vi "FdxCmdRxUDPControlCvi.vi"(8 "error in":errorcluster, 9 "UdpControl":T1={"UdpHandle"=0, "NetSelect"=3, "InterruptControl"=0} {"NetSelect" items=["FDX_RX_UDP_ONLY_A"=1, "FDX_RX_UDP_ONLY_B"=2, "FDX_RX_UDP_BOTH"=3]}, 11 "InstrumentHandle_port":u32) -> (0 "error out":errorcluster, 3 "InstrumentHandle_port":u32)   [LabVIEW 2020, in "AIM664LV.lvlib"]
doc: "This function allows to configure several settings of a UDP Receive Port"
uses:
  AIM664LV.lvlib
  AFDX_LibraryAdmin/FdxGlobalDllPath.vi
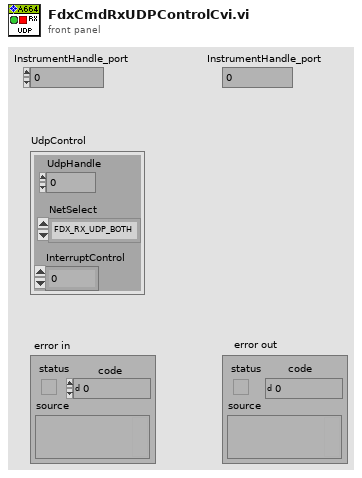
[diagram p1: front panel]
types:
  T1 = cluster{"UdpHandle":u32, "NetSelect":u32, "InterruptControl":u32}
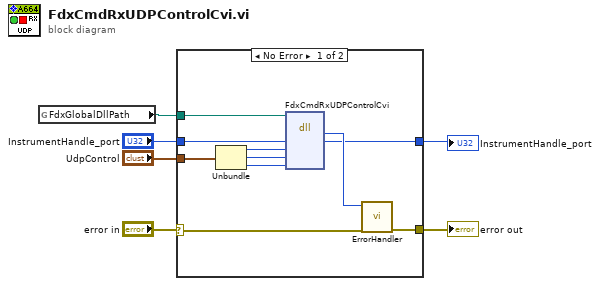
[diagram p0: block diagram]
diagram:
  n1 = global read "FdxGlobalDllPath.vi" "FdxGlobalDllPath"() -> (w4:path)
  n2 = case shown="No Error" "error in" {
    selector: "error in" -> [w15 w18]
    tunnel: [w16 w18] -> w6
    tunnel: w4 -> [w10 _]
    tunnel: "InstrumentHandle_port" -> [w9 w17]
    tunnel: [w8 w17] -> w2
    tunnel: "UdpControl" -> [w7 _]
    frame No Error {
      n3 = Unbundle(w7) -> ("UdpHandle"=w13:u32, "NetSelect"=w12:u32, "InterruptControl"=w11:u32)
      n4 = dll-call lib="aim_fdx.19.dll" fn="FdxCmdRxUDPControlCvi"(path in=w10, "InstrumentHandle"=w9, "UdpHandle"=w13, "NetSelect"=w12, "InterrupControl"=w11) -> ("status"=w14:i32, "InstrumentHandle"=w8:u32)  [unwired: 5 in, 2 out]
      n5 = call "ErrorHandler.vi"("error in"=w15, "AIM Error"=w14) -> ("error out"=w16:errorcluster)  [unwired: 9 in]
    }
    frame Error {
    }
  }
  "error out" <- w6
  "InstrumentHandle_port" <- w2
